vi "Choreo_TrajectorySwerve_SampleInternal.vi"(9 "TimeStamp":dbl, 11 "ChoreoTrajectorySwerve":T2) -> (3 "ChoreoSwerveSample":T1)   [LabVIEW 2019, in "ChoreoLib.lvlib"]
doc: "Internal routine to sample a swerve trajectory at a particular point in time.\n\nInputs:\n -- ChoreoTrajectorySwerve - cluster - data cluster for this trajectory \n -- timestamp - double - time to sample\n\nOutputs:\n -- ChoreoSwerveSample - cluster - interpolated sample"
uses:
  ChoreoLib.lvlib
  TypeDef/ChoreoTrajectorySwerve.ctl
  TypeDef/ChoreoSwerveSample.ctl
  TypeDef/ChoreoEventMarker.ctl
  <vilib>/Rock Robotics/WPI/ThirdParty/JAS_Junk/TrajLib/MathUtil_Interpolate.vi
  Choreo_SwerveSample_New.vi
  <vilib>/Rock Robotics/WPI/ThirdParty/JAS_Junk/TrajLib/MathUtil_Clamp.vi
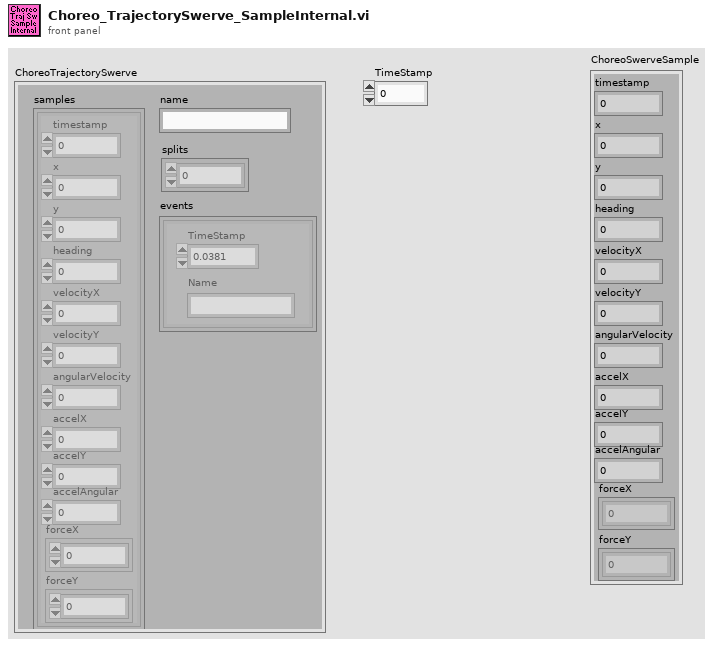
[diagram p1: front panel]
types:
  T1 = typedef "ChoreoLib.lvlib/ChoreoSwerveSample.ctl" = cluster{"timestamp":dbl, "x":dbl, "y":dbl, "heading":dbl, "velocityX":dbl, "velocityY":dbl, "angularVelocity":dbl, "accelX":dbl, "accelY":dbl, "accelAngular":dbl, "forceX":dbl[], "forceY":dbl[]}
  T2 = typedef "ChoreoLib.lvlib/ChoreoTrajectorySwerve.ctl" = cluster{"name":string, "samples":T1[], "splits":i32[], "events":T3[]}
  T3 = typedef "ChoreoLib.lvlib/ChoreoEventMarker.ctl" = cluster{"TimeStamp":dbl, "Name":string}
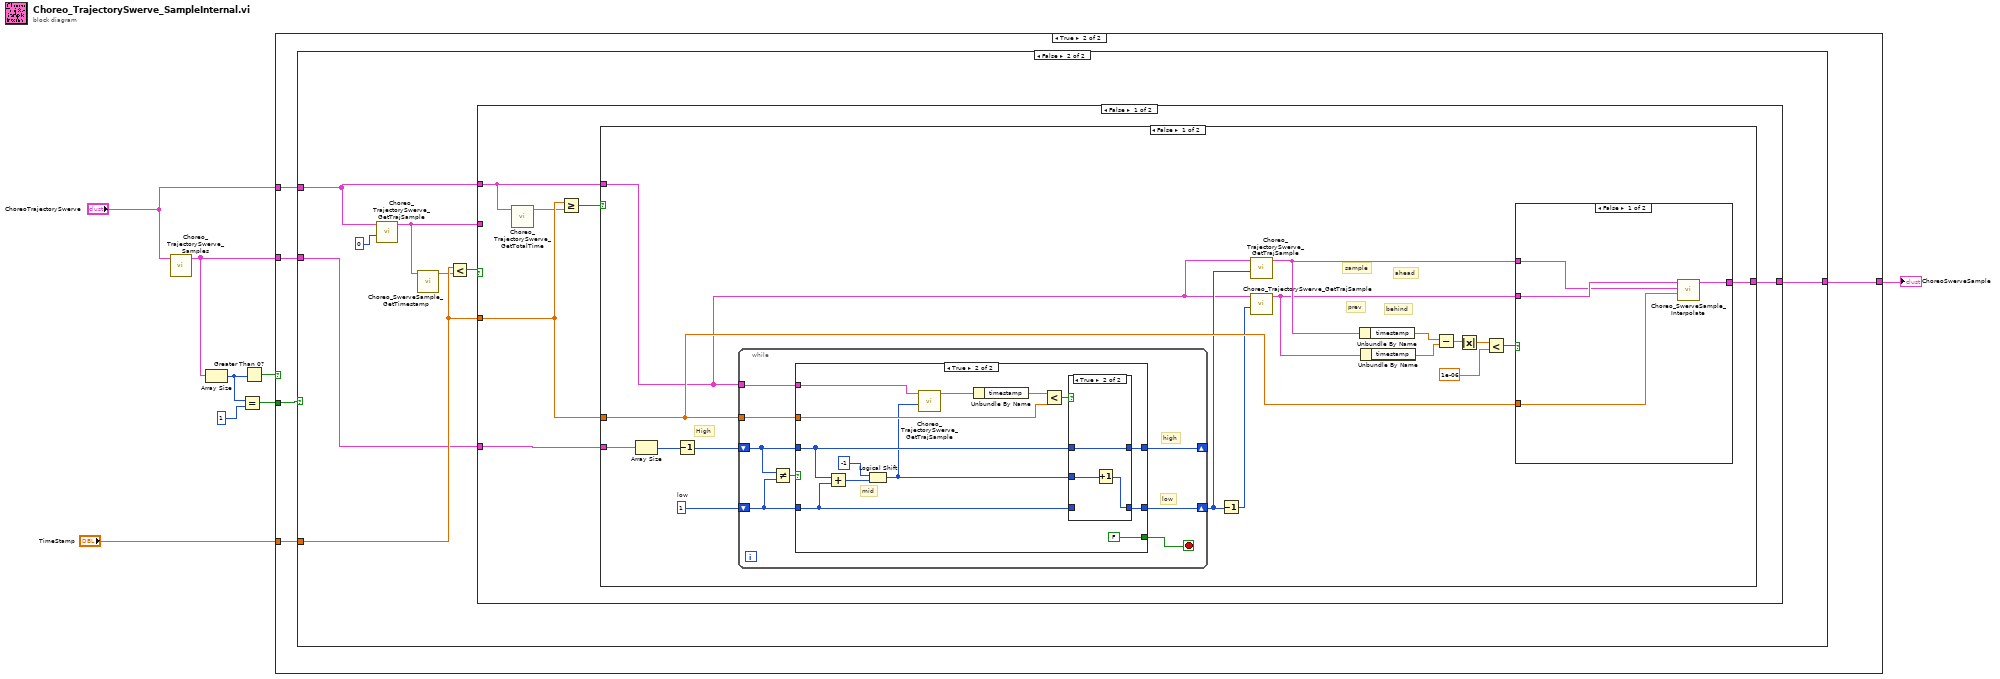
[diagram p0: block diagram]
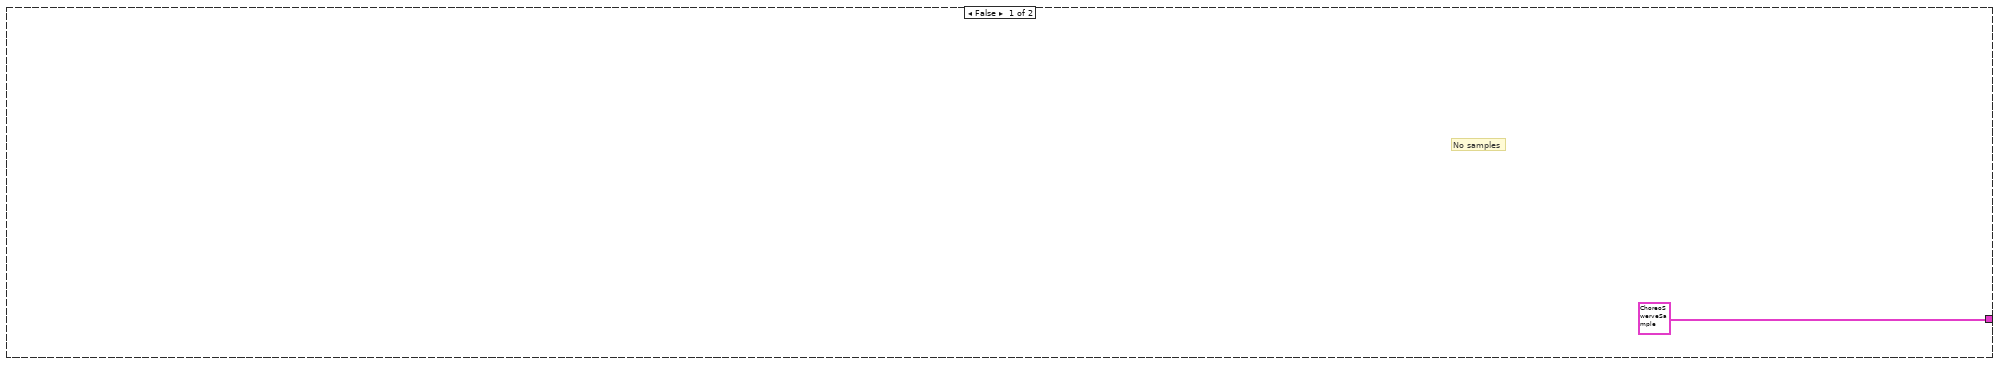
[diagram p2: hidden frame]
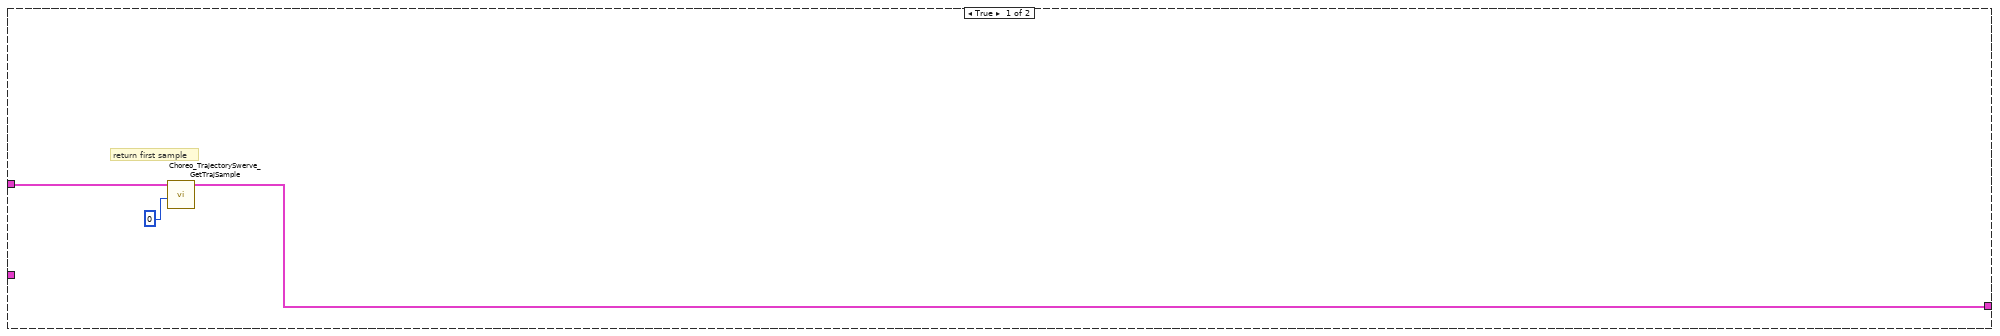
[diagram p3: hidden frame]
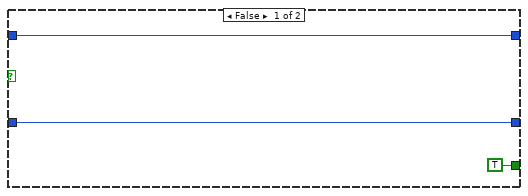
[diagram p5: hidden frame]
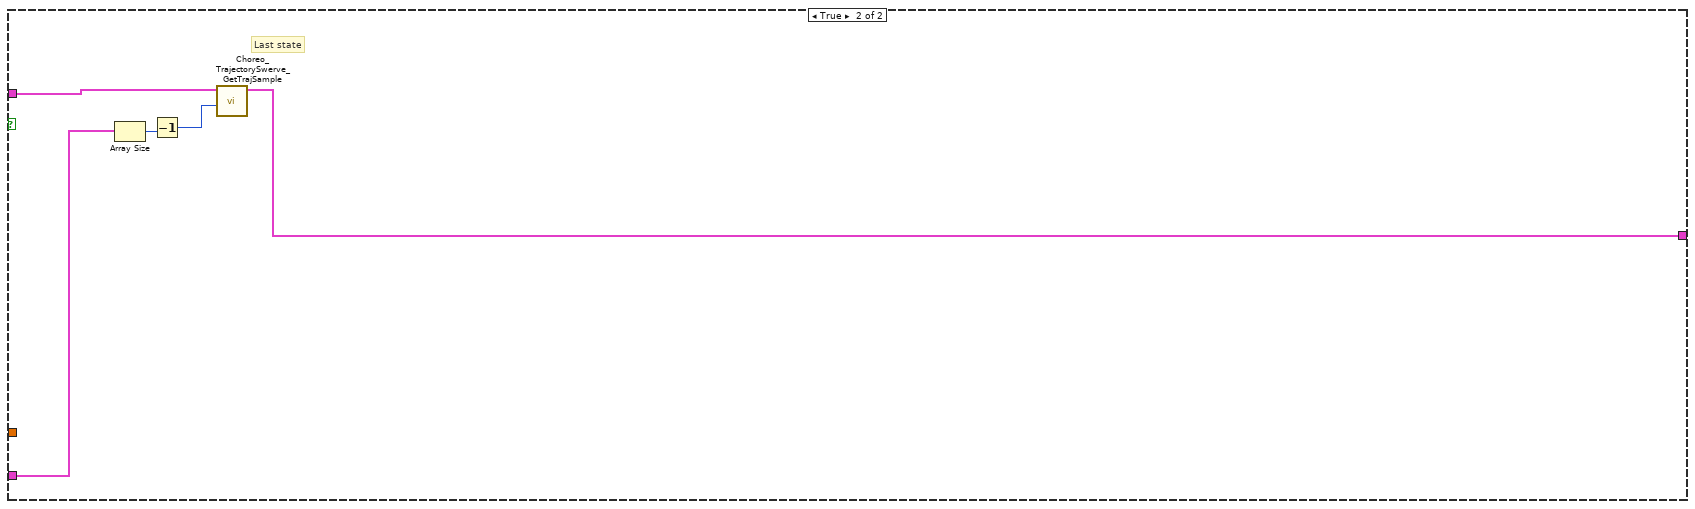
[diagram p7: hidden frame]
diagram:
  n1 = call "Choreo_TrajectorySwerve_Samples.vi"("ChoreoTrajectorySwerve"="ChoreoTrajectorySwerve") -> ("samples"=w2:T1[])  [unwired: 10 in]
  n2 = Array Size(array=w2) -> (size(s)=w5:i32)
  n3 = Equal?(x=w5, y=1) -> (x = y?=w3:bool)
  n4 = Greater Than 0?(x=w5) -> (x > 0?=w6:bool)
  n5 = case shown="True" w6 {
    tunnel: [T1 {"timestamp"=-999.0, "x"=0.0, "y"=0.0, "heading"=0.0, "velocityX"=0.0, "velocityY"=0.0, "angularVelocity"=0.0, "accelX"=0.0, "accelY"=0.0, "accelAngular"=0.0, "forceX"=[], "forceY"=[]} ("ChoreoSwerveSample") w14] -> w8
    tunnel: "TimeStamp" -> [_ w13]
    tunnel: w2 -> [_ w12]
    tunnel: w3 -> [_ w11]
    tunnel: "ChoreoTrajectorySwerve" -> [_ w10]
    frame False {
      # "No samples"
    }
    frame True {
      n6 = case shown="False" w11 {
        tunnel: [w16 w24] -> w14
        tunnel: w13 -> [_ w23]
        tunnel: w12 -> [_ w19]
        tunnel: w10 -> [w17 w18]
        frame True {
          # "return first sample"
          n7 = call "Choreo_TrajectorySwerve_GetTrajSample.vi"("index"=0, "ChoreoTrajectorySwerve"=w17) -> ("ChoreoSwerveSample"=w16:T1)  [unwired: 9 in]
        }
        frame False {
          n8 = call "Choreo_TrajectorySwerve_GetTrajSample.vi"("index"=0, "ChoreoTrajectorySwerve"=w18) -> ("ChoreoSwerveSample"=w21:T1)  [unwired: 9 in]
          n9 = call "Choreo_SwerveSample_GetTimestamp.vi"("ChoreoSwerveSample"=w21) -> ("Timestamp"=w20:dbl)  [unwired: 10 in]
          n10 = Less?(x=w23, y=w20) -> (x < y?=w25:bool)
          n11 = case shown="False" w25 {
            tunnel: w21 -> [_ w88]
            tunnel: [w30 w88] -> w24
            tunnel: w18 -> [w28 _]
            tunnel: w23 -> [w29 _]
            tunnel: w19 -> [w26 _]
            frame False {
              n12 = call "Choreo_TrajectorySwerve_GetTotalTime.vi"("ChoreoTrajectorySwerve"=w28) -> ("TotalTime"=w27:dbl)  [unwired: 10 in]
              n13 = Greater Or Equal?(x=w29, y=w27) -> (x >= y?=w31:bool)
              n14 = case shown="False" w31 {
                tunnel: [w41 w84] -> w30
                tunnel: w28 -> [w32 w85]
                tunnel: w29 -> [w39 _]
                tunnel: w26 -> [w33 w83]
                frame False {
                  w46 = 1  # low
                  # "ahead"
                  # "behind"
                  # "prev"
                  # "sample"
                  # "High"
                  n15 = Array Size(array=w33) -> (size(s)=w48:i32)
                  n16 = Decrement(x=w48) -> (x-1=w47:i32)
                  n17 = while {
                    shift-right: [w59] -> w37
                    shift-left: w46 -> [w55]
                    shift-right: [w60] -> _
                    shift-left: w47 -> [w56]
                    tunnel: w32 -> [w58]
                    tunnel: w39 -> [w61]
                    stop <- w54 stop-if-true
                    # "high"
                    # "low"
                    n18 = Not Equal?(x=w56, y=w55) -> (x != y?=w57:bool)
                    n19 = case shown="True" w57 {
                      tunnel: w61 -> [_ w74]
                      tunnel: w56 -> [w64 w72]
                      tunnel: w55 -> [w63 w71]
                      tunnel: [w64 w70] -> w60
                      tunnel: [w63 w69] -> w59
                      tunnel: w58 -> [_ w66]
                      tunnel: [TRUE FALSE] -> w54
                      frame False {
                      }
                      frame True {
                        # "mid"
                        n20 = Add(x=w72, y=w71) -> (x+y=w77:i32)
                        n21 = Logical Shift(y=i16 -1, x=w77) -> (x << y=w67:i32)
                        n22 = call "Choreo_TrajectorySwerve_GetTrajSample.vi"("index"=w67, "ChoreoTrajectorySwerve"=w66) -> ("ChoreoSwerveSample"=w65:T1)  [unwired: 9 in]
                        n23 = Unbundle By Name(w65) -> ("timestamp"=w75:dbl)
                        n24 = Less?(x=w75, y=w74) -> (x < y?=w73:bool)
                        n25 = case shown="True" w73 {
                          tunnel: w72 -> [_ w82]
                          tunnel: [w78 w82] -> w70
                          tunnel: w67 -> [w78 w81]
                          tunnel: w71 -> [w79 _]
                          tunnel: [w79 w80] -> w69
                          frame False {
                          }
                          frame True {
                            n26 = Increment(x=w81) -> (x+1=w80:i32)
                          }
                        }
                      }
                    }
                  }
                  n27 = Decrement(x=w37) -> (x-1=w36:i32)
                  n28 = call "Choreo_TrajectorySwerve_GetTrajSample.vi"("index"=w37, "ChoreoTrajectorySwerve"=w32) -> ("ChoreoSwerveSample"=w35:T1)  [unwired: 9 in]
                  n29 = call "Choreo_TrajectorySwerve_GetTrajSample.vi"("index"=w36, "ChoreoTrajectorySwerve"=w32) -> ("ChoreoSwerveSample"=w34:T1)  [unwired: 9 in]
                  n30 = Unbundle By Name(w35) -> ("timestamp"=w38:dbl)
                  n31 = Unbundle By Name(w34) -> ("timestamp"=w40:dbl)
                  n32 = Subtract(x=w38, y=w40) -> (x-y=w45:dbl)
                  n33 = Absolute Value(x=w45) -> (abs(x)=w44:dbl)
                  n34 = Less?(x=w44, y=1e-06) -> (x < y?=w42:bool)
                  n35 = case shown="False" w42 {
                    tunnel: w35 -> [w50 w53]
                    tunnel: [w49 w53] -> w41
                    tunnel: w34 -> [w51 _]
                    tunnel: w39 -> [w52 _]
                    frame False {
                      n36 = call "Choreo_SwerveSample_Interpolate.vi"("TimeStamp"=w52, "endValueSample"=w50, "ChoreoSwerveSample"=w51) -> ("InterpolatedSample"=w49:T1)  [unwired: 8 in]
                    }
                    frame True {
                    }
                  }
                }
                frame True {
                  # "Last state"
                  n37 = Array Size(array=w83) -> (size(s)=w87:i32)
                  n38 = Decrement(x=w87) -> (x-1=w86:i32)
                  n39 = call "Choreo_TrajectorySwerve_GetTrajSample.vi"("index"=w86, "ChoreoTrajectorySwerve"=w85) -> ("ChoreoSwerveSample"=w84:T1)  [unwired: 9 in]
                }
              }
            }
            frame True {
              # "First State"
            }
          }
        }
      }
    }
  }
  "ChoreoSwerveSample" <- w8
